vi "Controller Process.vi"(8 "error in (no error)":errorcluster, 11 "View Model":T1) -> (0 "error out":errorcluster)   [LabVIEW 2017]
uses:
  View Model/Controls/View Model.ctl
  Error Handler/Controls/Error Model.ctl
  Error Handler/Controls/Error Data.ctl
  Error Handler/Controls/Error Type.ctl
  View Model/Controls/Shared Model.ctl
  Configuration/Controls/Config Model.ctl
  Configuration/Controls/Config CMD.ctl
  Configuration/Controls/Config Data.ctl
  Controls/Controller Model.ctl
  Controls/Controller Overhead.ctl
  Controls/Controller States.ctl
  Controls/Controller Message Data.ctl
  Controls/Controller Message Name.ctl
  Controls/Controller CMD.ctl
  Views/User Console View/Controls/User Console - Transaction Enum.ctl
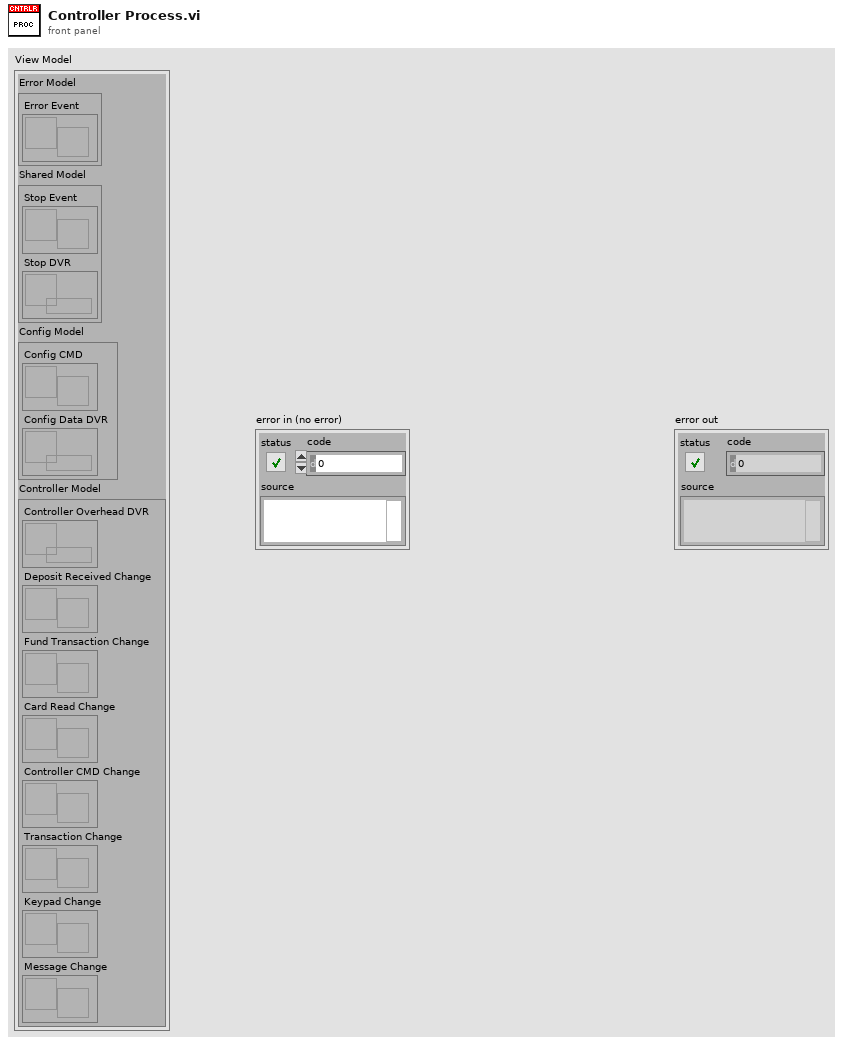
[diagram p1: front panel]
types:
  T1 = typedef "View Model.ctl" = cluster{"Error Model":T2, "Shared Model":T3, "Config Model":T4, "Controller Model":T5}
  T2 = typedef "Error Model.ctl" = cluster{"Error Event":refnum<user-event>}
  T3 = typedef "Shared Model.ctl" = cluster{"Stop Event":refnum<user-event>, "Stop DVR":refnum<data-value>}
  T4 = typedef "Config Model.ctl" = cluster{"Config CMD":refnum<user-event>, "Config Data DVR":refnum<data-value>}
  T5 = typedef "Controller Model.ctl" = cluster{"Controller Overhead DVR":refnum<data-value>, "Deposit Received Change":refnum<user-event>, "Fund Transaction Change":refnum<user-event>, "Card Read Change":refnum<user-event>, "Controller CMD Change":refnum<user-event>, "Transaction Change":refnum<user-event>, "Keypad Change":refnum<user-event>, "Message Change":refnum<user-event>}
  T6 = typedef "Controller States.ctl" = enum16{"Idle", "Init", "Display Message", "Login", "Balance Inquiry", "Deposit", "Withdrawal", "Fast Cash", "Terminate"}
  T7 = typedef "User Console - Transaction Enum.ctl" = enum16{"Balance Inquiry", "Deposit", "Withdrawal", "Fat Cash", "New Transaction", "Terminate Session"}
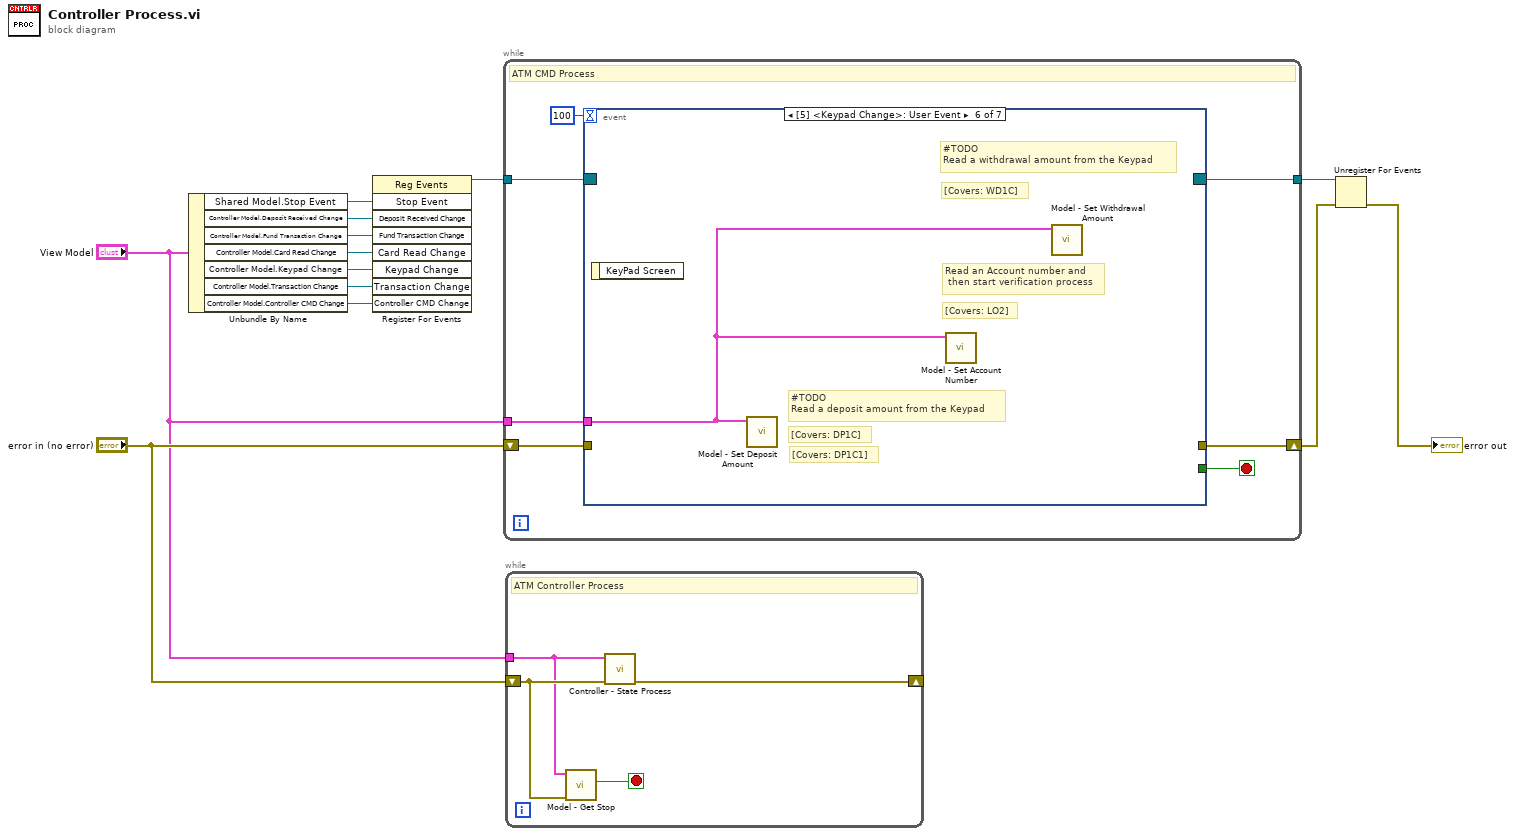
[diagram p0: block diagram]
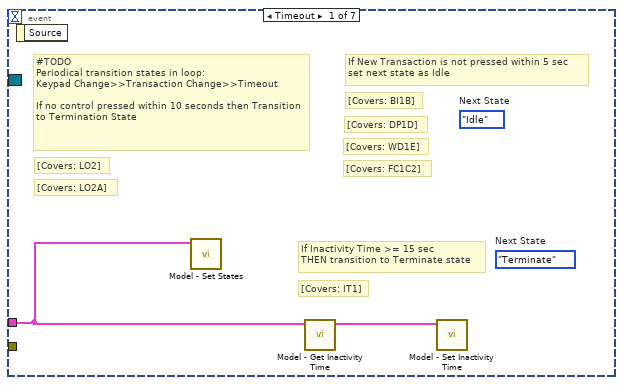
[diagram p2: hidden frame]
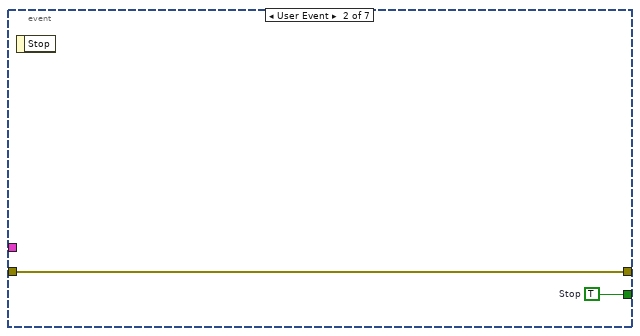
[diagram p3: hidden frame]
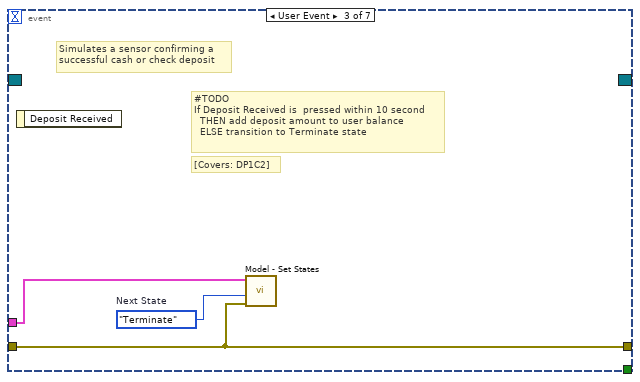
[diagram p4: hidden frame]
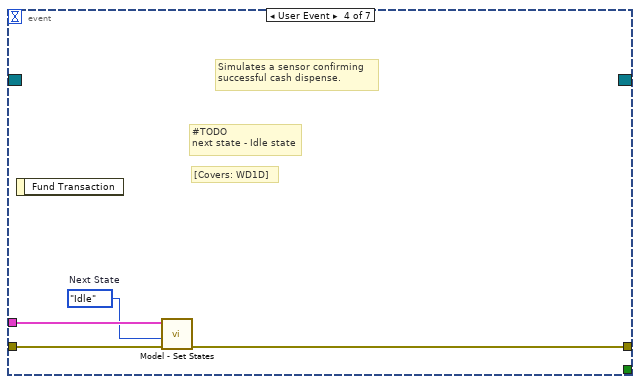
[diagram p5: hidden frame]
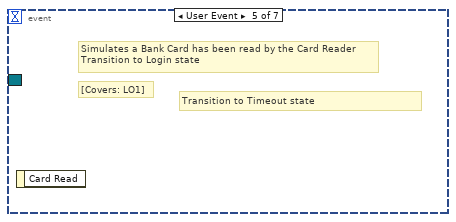
[diagram p6: hidden frame]
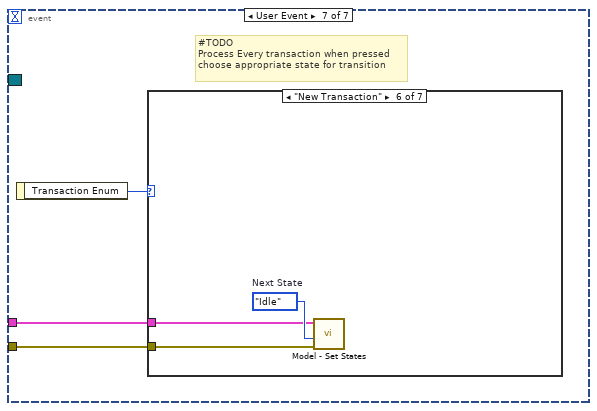
[diagram p7: hidden frame]
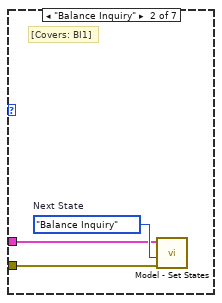
[diagram p9: hidden frame]
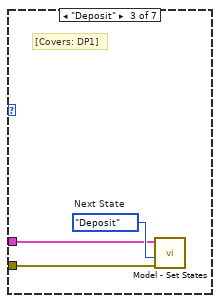
[diagram p10: hidden frame]
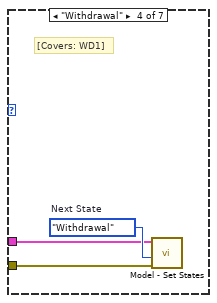
[diagram p11: hidden frame]
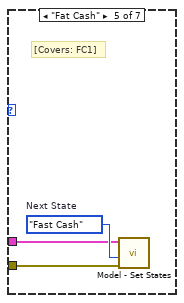
[diagram p12: hidden frame]
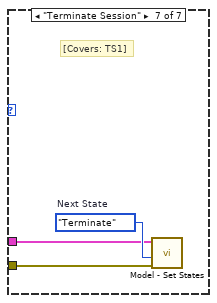
[diagram p13: hidden frame]
diagram:
  n1 = Unbundle By Name("View Model") -> ("Shared Model.Stop Event"=w13:refnum<user-event>, "Controller Model.Deposit Received Change"=w8:refnum<user-event>, "Controller Model.Fund Transaction Change"=w7:refnum<user-event>, "Controller Model.Card Read Change"=w6:refnum<user-event>, "Controller Model.Keypad Change"=w5:refnum<user-event>, "Controller Model.Transaction Change"=w4:refnum<user-event>, "Controller Model.Controller CMD Change"=w3:refnum<user-event>)
  n2 = register-events(w13, w8, w7, w6, w5, w4, w3) -> (reference out=w12:refnum<event-registration>)  [unwired: 2 in, 1 out]
  n3 = while {
    tunnel: w12 -> [w20]
    shift-right: [w17] -> w10
    shift-left: "error in (no error)" -> [w18]
    tunnel: [w16] -> w11
    tunnel: "View Model" -> [w14]
    stop <- w19 stop-if-true
    # "ATM CMD Process"
    n4 = event shown="[5] <Keypad Change>: User Event" {
      selector: w20 -> [_ _ _ _ _ _ _]
      dyn-events: [_ _ _ _ _ _ _] -> w16
      timeout: 100 -> [_ _ _ _ _ _ _]
      tunnel: [_ w24 _ _ _ _ _] -> w19
      tunnel: w18 -> [_ w23 w26 w31 _ _ w33]
      tunnel: [_ w23 w26 w28 _ _ _] -> w17
      tunnel: w14 -> [w22 _ w27 w30 _ w32 w34]
      event Timeout {
        (unwired) Controller_States."Terminate"  # Next State
        (unwired) Controller_States."Idle"  # Next State
        # "[Covers: IT1]"
        # "If Inactivity Time >= 15 sec \nTHEN transition to Terminate state"
        # "[Covers: FC1C2]"
        # "[Covers: WD1E]"
        # "[Covers: DP1D]"
        # "[Covers: BI1B]"
        # "If New Transaction is not pressed within 5 sec\nset next state as Idle"
        # "[Covers: LO2A]"
        # "[Covers: LO2]"
        # "#TODO\nPeriodical transition states in loop:\nKeypad Change>>Transaction Change>>Timeout\n\nIf no control pressed within 10 seconds then Transition to Termination State"
        n5 = event-data() -> ()  [unwired: 1 in, 1 out]
        n6 = call "Model - Set States.vi"("View Model"=w22) -> ()  [unwired: 9 in, 2 out]
        n7 = call "Model - Get Inactivity Time.vi"("View Model"=w22) -> ("View Model"=w21:T1)  [unwired: 8 in, 2 out]
        n8 = call "Model - Set Inactivity Time.vi"("View Model"=w21) -> ()  [unwired: 9 in, 2 out]
      }
      event User Event {
        w24 = TRUE  # Stop
        n9 = event-data() -> ()  [unwired: 1 in, 1 out]
      }
      event User Event {
        w25 = Controller_States."Terminate"  # Next State
        # "[Covers: DP1C2]"
        # "#TODO\nIf Deposit Received is  pressed within 10 second\n  THEN add deposit amount to user balance\n  ELSE transition to Terminate state"
        # "Simulates a sensor confirming a\nsuccessful cash or check deposit"
        n10 = event-data() -> ()  [unwired: 1 in, 1 out]
        n11 = call "Model - Set States.vi"("error in (no error)"=w26, "Next State"=w25, "View Model"=w27) -> ()  [unwired: 7 in, 2 out]
      }
      event User Event {
        w29 = Controller_States."Idle"  # Next State
        # "[Covers: WD1D]"
        # "#TODO\nnext state - Idle state"
        # "Simulates a sensor confirming\nsuccessful cash dispense."
        n12 = event-data() -> ()  [unwired: 1 in, 1 out]
        n13 = call "Model - Set States.vi"("error in (no error)"=w31, "Next State"=w29, "View Model"=w30) -> ("error out"=w28:errorcluster)  [unwired: 7 in, 1 out]
      }
      event User Event {
        # "Transition to Timeout state"
        # "[Covers: LO1]"
        # "Simulates a Bank Card has been read by the Card Reader\nTransition to Login state"
        n14 = event-data() -> ()  [unwired: 1 in, 1 out]
      }
      event User Event {
        # "[Covers: WD1C]"
        # "#TODO\nRead a withdrawal amount from the Keypad"
        # "[Covers: DP1C1]"
        # "[Covers: DP1C]"
        # "#TODO\nRead a deposit amount from the Keypad"
        # "[Covers: LO2]"
        # "Read an Account number and\n then start verification process"
        n15 = event-data() -> ()  [unwired: 1 in, 1 out]
        n16 = call "Model - Set Deposit Amount.vi"("View Model"=w32) -> ()  [unwired: 9 in, 2 out]
        n17 = call "Model - Set Account Number.vi"("View Model"=w32) -> ()  [unwired: 9 in, 2 out]
        n18 = call "Model - Set Withdrawal Amount.vi"("View Model"=w32) -> ()  [unwired: 9 in, 2 out]
      }
      event User Event {
        # "#TODO\nProcess Every transaction when pressed\nchoose appropriate state for transition"
        n19 = event-data() -> ("Transaction Enum"=w35:T7)  [unwired: 1 in]
        n20 = case shown="\"New Transaction\"" w35 {
          tunnel: w34 -> [_ w37 w39 w43 w46 w49 w52]
          tunnel: w33 -> [_ w36 w40 w42 w45 w48 w51]
          frame Default {
          }
          frame "Balance Inquiry" {
            w38 = Controller_States."Balance Inquiry"  # Next State
            # "[Covers: BI1]"
            n21 = call "Model - Set States.vi"("error in (no error)"=w36, "Next State"=w38, "View Model"=w37) -> ()  [unwired: 7 in, 2 out]
          }
          frame "Deposit" {
            w41 = Controller_States."Deposit"  # Next State
            # "[Covers: DP1]"
            n22 = call "Model - Set States.vi"("error in (no error)"=w40, "Next State"=w41, "View Model"=w39) -> ()  [unwired: 7 in, 2 out]
          }
          frame "Withdrawal" {
            w44 = Controller_States."Withdrawal"  # Next State
            # "[Covers: WD1]"
            n23 = call "Model - Set States.vi"("error in (no error)"=w42, "Next State"=w44, "View Model"=w43) -> ()  [unwired: 7 in, 2 out]
          }
          frame "Fat Cash" {
            w47 = Controller_States."Fast Cash"  # Next State
            # "[Covers: FC1]"
            n24 = call "Model - Set States.vi"("error in (no error)"=w45, "Next State"=w47, "View Model"=w46) -> ()  [unwired: 7 in, 2 out]
          }
          frame "New Transaction" {
            w50 = Controller_States."Idle"  # Next State
            n25 = call "Model - Set States.vi"("error in (no error)"=w48, "Next State"=w50, "View Model"=w49) -> ()  [unwired: 7 in, 2 out]
          }
          frame "Terminate Session" {
            w53 = Controller_States."Terminate"  # Next State
            # "[Covers: TS1]"
            n26 = call "Model - Set States.vi"("error in (no error)"=w51, "Next State"=w53, "View Model"=w52) -> ()  [unwired: 7 in, 2 out]
          }
        }
      }
    }
  }
  n27 = while {
    tunnel: "View Model" -> [w55]
    shift-right: [w54] -> _
    shift-left: "error in (no error)" -> [w56]
    stop <- w57 stop-if-true
    # "ATM Controller Process"
    n28 = call "Model - Get Stop.vi"("error in (no error)"=w56, "View Model"=w55) -> ("Stop"=w57:bool)  [unwired: 7 in, 2 out]
    n29 = call "Controller - State Process.vi"("error in (no error)"=w56, "View Model"=w55) -> ("error out"=w54:errorcluster)  [unwired: 8 in, 1 out]
  }
  n30 = Unregister For Events(event registration refnum=w11, error in=w10) -> (error out=→"error out":errorcluster)
